vi "Production Mode.vi"() -> ()   [LabVIEW 2019]
uses:
  <vilib>/Instr/_visa.llb/VISA Configure Serial Port (Instr).vi
  <vilib>/regexp/Match Regular Expression.xnode
panel:
  in  "Name":string
  in  "sMDT Code":string
  out "Previous\nTest Passed":bool
  out "Status":string
  in  "Start":bool
  out "Leak":string
  out "Pressure (mTorr)":dbl
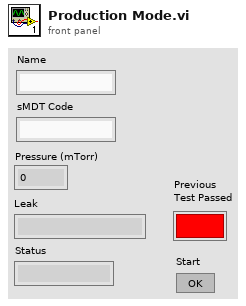
[diagram p1: front panel]
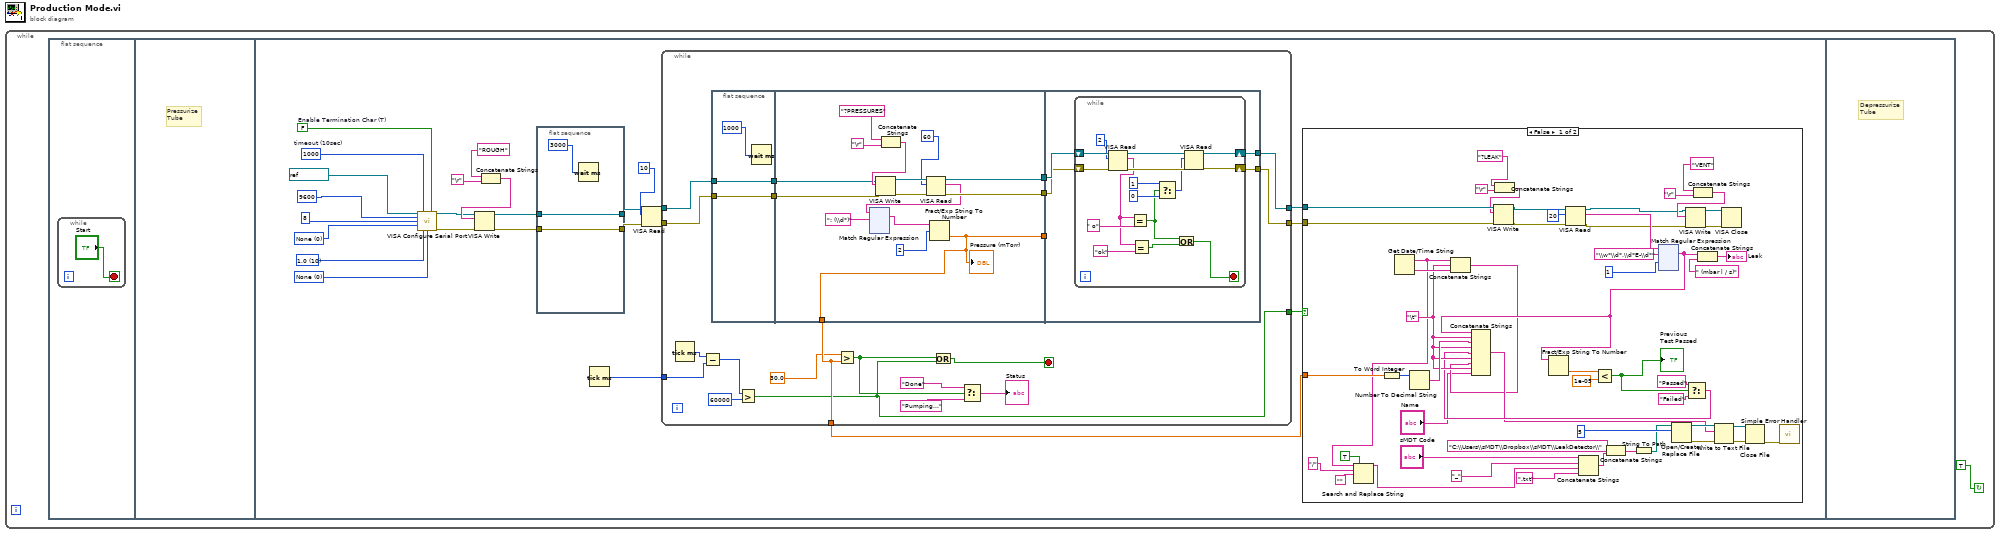
[diagram p0: block diagram]
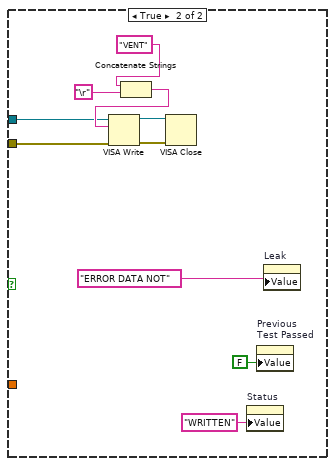
[diagram p2: hidden frame]
diagram:
  n1 = while {
    stop <- TRUE continue-if-true
    n2 = flat-sequence {
      frame #0 {
        n3 = while {
          stop <- "Start" stop-if-true
        }
      }
      frame #1 {
        # "Pressurize\nTube"
      }
      frame #2 {
        w21 = u16 0 items=["None"=0, "XON/XOFF"=1, "RTS/CTS"=2, "DTR/DSR"=4] ("flow control")
        w22 = u16 10 items=["1.0"=10, "1.5"=15, "2.0"=20] ("stop bits")
        w23 = u16 0 items=["None", "Odd", "Even", "Mark", "Space"] ("parity")
        w26 = FALSE  # Enable Termination Char (T)
        w27 = u32 1000  # timeout (10sec)
        n4 = call-poly "VISA Configure Serial Port"("VISA resource name"=refnum<visa-resource-name> "COM3", "timeout (10sec)"=w27, "Enable Termination\nChar (T)"=w26, "baud rate (9600)"=u32 9600 ("baud rate"), "data bits (8)"=u16 8 ("data bits"), "parity (0:none)"=w23, "stop bits (10: 1 bit)"=w22, "flow control (0:none)"=w21) -> ("VISA resource name out"=w6:refnum<visa-resource-name>, "error out"=w5:errorcluster)  [unwired: 6 in]
        n5 = Concatenate Strings("ROUGH", "\r") -> (w18:string)
        n6 = VISA Write(VISA resource name=w6, write buffer=w18, error in (no error)=w5) -> (VISA resource name out=w17:refnum<visa-resource-name>, error out=w16:errorcluster)  [unwired: 1 out]
        n7 = flat-sequence {
          tunnel: w17 -> [w378]
          tunnel: w16 -> [w379]
          tunnel: [w379] -> w13
          tunnel: [w378] -> w14
          frame #0 {
            n8 = Wait (ms)(milliseconds to wait=3000) -> ()  [unwired: 1 out]
          }
        }
        n9 = Tick Count (ms)() -> (millisecond timer value=w3:u32)
        n10 = VISA Read(VISA resource name=w14, byte count=10, error in (no error)=w13) -> (VISA resource name out=w11:refnum<visa-resource-name>, error out=w12:errorcluster)  [unwired: 2 out]
        n11 = while {
          tunnel: w11 -> [w225]
          tunnel: w12 -> [w224]
          tunnel: [w214] -> w10
          tunnel: [w213] -> w9
          tunnel: [w218] -> w7
          tunnel: [w209] -> w4
          tunnel: w3 -> [w207]
          stop <- w210 stop-if-true
          n12 = Tick Count (ms)() -> (millisecond timer value=w208:u32)
          n13 = Subtract(x=w208, y=w207) -> (x-y=w206:u32)
          n14 = flat-sequence {
            tunnel: w225 -> [w228]
            tunnel: w224 -> [w227]
            tunnel: [w228] -> w223
            tunnel: [w227] -> w222
            tunnel: w223 -> [w237]
            tunnel: w222 -> [w236]
            tunnel: [w230] -> w218
            tunnel: [w234] -> w217
            tunnel: [w235] -> w216
            tunnel: [w230] -> w215
            tunnel: w217 -> [w360]
            tunnel: w216 -> [w361]
            tunnel: w215 -> [_]
            tunnel: [w359] -> w214
            tunnel: [w358] -> w213
            frame #0 {
              n15 = Wait (ms)(milliseconds to wait=1000) -> ()  [unwired: 1 out]
            }
            frame #1 {
              n16 = Concatenate Strings("?PRESSURES", "\r") -> (w238:string)
              n17 = VISA Write(VISA resource name=w237, write buffer=w238, error in (no error)=w236) -> (VISA resource name out=w243:refnum<visa-resource-name>, error out=w242:errorcluster)  [unwired: 1 out]
              n18 = VISA Read(VISA resource name=w243, byte count=60, error in (no error)=w242) -> (VISA resource name out=w235:refnum<visa-resource-name>, read buffer=w229:string, error out=w234:errorcluster)  [unwired: 1 out]
              n19 = xnode "Match Regular Expression"("input string"=w229, "regular expression"=": (\\d*)") -> ("whole match"=w233:string)  [unwired: 4 in, 4 out]
              n20 = Fract/Exp String To Number(string=w233, offset=2) -> (number=w230:dbl)  [unwired: 2 in, 1 out]
              "Pressure (mTorr)" <- w230
            }
            frame #2 {
              n21 = while {
                shift-right: [w371] -> w359
                shift-left: w361 -> [w377]
                shift-right: [w372] -> w358
                shift-left: w360 -> [w374]
                stop <- w362 stop-if-true
                n22 = VISA Read(VISA resource name=w377, byte count=2, error in (no error)=w374) -> (VISA resource name out=w375:refnum<visa-resource-name>, read buffer=w365:string, error out=w373:errorcluster)  [unwired: 1 out]
                n23 = Equal?(x=w365, y=" o") -> (x = y?=w363:bool)
                n24 = Equal?(x=w365, y="ok") -> (x = y?=w364:bool)
                n25 = Select(t=1, s=w363, f=0) -> (s? t:f=w368:i32)
                n26 = Or(x=w363, y=w364) -> (x .or. y?=w362:bool)
                n27 = VISA Read(VISA resource name=w375, byte count=w368, error in (no error)=w373) -> (VISA resource name out=w371:refnum<visa-resource-name>, error out=w372:errorcluster)  [unwired: 2 out]
              }
            }
          }
          n28 = Greater?(x=w206, y=u32 60000) -> (0:w209:bool)
          n29 = Greater?(x=30.0 ("Pump Pressure"), y=w218) -> (0:w211:bool)
          n30 = Or(x=w211, y=w209) -> (x .or. y?=w210:bool)
          n31 = Select(t="Done", s=w211, f="Pumping...") -> (s? t:f=→"Status":string)
        }
        n32 = case shown="False" w4 {
          tunnel: w10 -> [w67 w199]
          tunnel: w9 -> [w66 w198]
          tunnel: w7 -> [w44 _]
          frame False {
            w38 = "\t"
            n33 = To Word Integer(number=w44) -> (16bit integer=w43:i16)
            n34 = Get Date/Time String() -> (date string=w32:string, time string=w42:string)  [unwired: 3 in]
            n35 = Search and Replace String(replace all?=TRUE, input string=w32, search string="/", replace string="") -> (result string=w28:string)  [unwired: 4 in, 3 out]
            n36 = Number To Decimal String(number=w43) -> (decimal integer string=w39:string)  [unwired: 1 in]
            n37 = Concatenate Strings(w32, w38, w42) -> (w35:string)
            n38 = Concatenate Strings("?LEAK", "\r") -> (w63:string)
            n39 = VISA Write(VISA resource name=w67, write buffer=w63, error in (no error)=w66) -> (VISA resource name out=w62:refnum<visa-resource-name>, error out=w61:errorcluster)  [unwired: 1 out]
            n40 = VISA Read(VISA resource name=w62, byte count=20, error in (no error)=w61) -> (VISA resource name out=w69:refnum<visa-resource-name>, read buffer=w70:string, error out=w68:errorcluster)  [unwired: 1 out]
            n41 = Concatenate Strings("sMDT Code", "_", w28, ".txt") -> (w50:string)
            n42 = Concatenate Strings("C:\\Users\\sMDT\\Dropbox\\sMDT\\LeakDetector\\", w50) -> (w33:string)
            n43 = String To Path(string=w33) -> (path=w52:path)
            n44 = xnode "Match Regular Expression"("input string"=w70, "regular expression"="\\w*\\d*.\\d*E-\\d*", "offset (0)"=1) -> ("whole match"=w47:string)  [unwired: 3 in, 4 out]
            n45 = Fract/Exp String To Number(string=w47) -> (number=w59:dbl)  [unwired: 3 in, 1 out]
            n46 = Less?(x=w59, y=1e-05) -> (x < y?=w45:bool)
            "Previous\nTest Passed" <- w45
            n47 = Open/Create/Replace File(file path (use dialog)=w52, operation (0:open)=5) -> (refnum out=w57:refnum<file>, error out=w55:errorcluster)  [unwired: 4 in, 1 out]
            n48 = Select(t="Passed", s=w45, f="Failed") -> (s? t:f=w37:string)
            n49 = Concatenate Strings(w47, w38, w39, w38, w37, w38, w35, w38, "Name") -> (w36:string)
            n50 = Concatenate Strings("VENT", "\r") -> (w78:string)
            n51 = VISA Write(VISA resource name=w69, write buffer=w78, error in (no error)=w68) -> (VISA resource name out=w77:refnum<visa-resource-name>, error out=w76:errorcluster)  [unwired: 1 out]
            n52 = Concatenate Strings(w47, " (mbar l / s)") -> (→"Leak":string)
            n53 = Write to Text File(file (use dialog)=w57, text=w36, error in=w55) -> (refnum out=w56:refnum<file>, error out=w54:errorcluster)  [unwired: 1 in, 1 out]
            n54 = VISA Close(VISA resource name=w77, error in (no error)=w76) -> ()  [unwired: 1 out]
            n55 = Close File(refnum=w56, error in=w54) -> (error out=w53:errorcluster)  [unwired: 1 out]
            n56 = call <vilib>:"Simple Error Handler.vi"("error in (no error)"=w53) -> ()  [unwired: 4 in, 5 out]
          }
          frame True {
            n57 = Concatenate Strings("VENT", "\r") -> (w202:string)
            n58 = VISA Write(VISA resource name=w199, write buffer=w202, error in (no error)=w198) -> (VISA resource name out=w203:refnum<visa-resource-name>, error out=w204:errorcluster)  [unwired: 1 out]
            n59 = VISA Close(VISA resource name=w203, error in (no error)=w204) -> ()  [unwired: 1 out]
            n60 = property on="Status" class="Str"("Value"="WRITTEN" ("Status")) -> ()  [unwired: 2 in, 2 out]
            n61 = property on="Previous\nTest Passed" class="Bool (strict)"("Value"=FALSE ("Previous\nTest Passed")) -> ()  [unwired: 2 in, 2 out]
            n62 = property on="Leak" class="Str"("Value"="ERROR DATA NOT") -> ()  [unwired: 2 in, 2 out]
          }
        }
      }
      frame #3 {
        # "Depressurize\nTube"
      }
    }
  }
